vi "Inspect Update Global Variables.vi"(11 "Mode":enum16{"Start", "End"}(ring)) -> ()   [LabVIEW 2019]
uses:
  Common.llb/IVB Variable Data Cluster.ctl
  <vilib>/vision/Image Controls.llb/IMAQ Image.ctl
  Common.llb/IVB Global Variable - Manager Mode.ctl
  Common.llb/IVB Measure ID.ctl
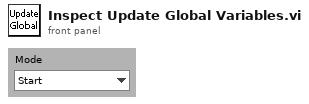
[diagram p1: front panel]
types:
  T1 = typedef "IVB Variable Data Cluster.ctl" = cluster{"String":string, "Numeric":dbl, "Boolean":bool, "Point":cluster{"X":dbl, "Y":dbl}, "Image":T2, "1D String":string[], "1D Numeric":dbl[], "1D Boolean":bool[]}
  T2 = typedef "IMAQ Image.ctl" = refnum<image>
  T3 = typedef "IVB Measure ID.ctl" = cluster{"Step GUID":string, "Result GUID":string, "Index":i32}
  T4 = typedef "IVB Global Variable - Manager Mode.ctl" = enum16{"Init", "Delete User Defined", "Update User Defined", "Get All User Defined", "Get All System", "Set Current Value System", "Set Current Value User Defined", "Add/Update Variable"}
  T5 = enum16{"Reset", "Start Process", "Suspend Process", "Add Elapsed Time", "Get Results"}
  T6 = cluster{"Numeric":dbl, "Boolean":bool, "String":string, "1D Numeric":dbl[], "1D Boolean":bool[], "1D String":string[]}
  T7 = cluster{"Active Time":dbl, "Idle Time":dbl, "Ratio Active/Total":dbl}
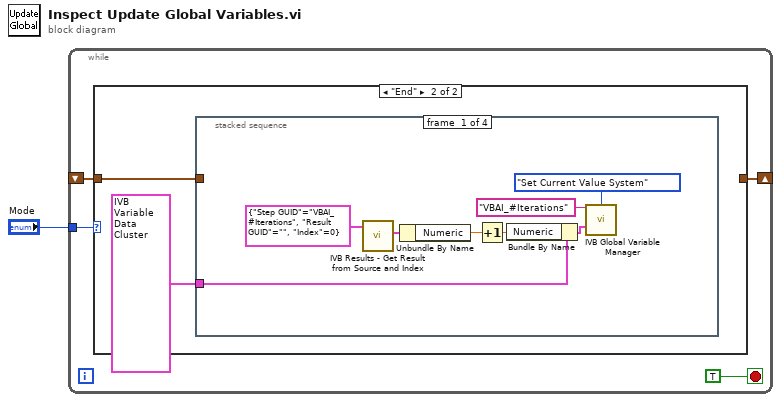
[diagram p0: block diagram]
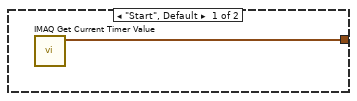
[diagram p2: hidden frame]
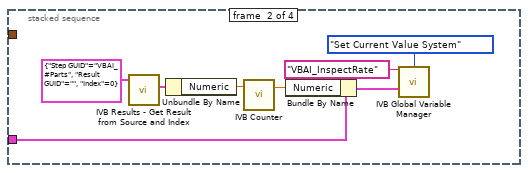
[diagram p3: hidden frame]
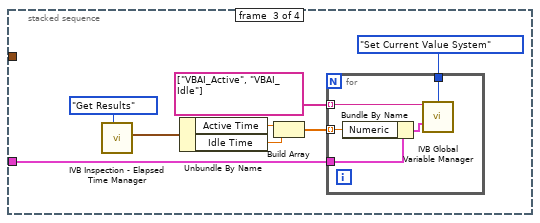
[diagram p4: hidden frame]
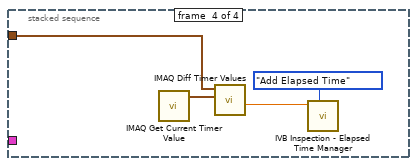
[diagram p5: hidden frame]
diagram:
  n1 = while {
    tunnel: "Mode" -> [w5]
    shift-right: [w4] -> _
    shift-left: _ -> [w3]
    stop <- TRUE stop-if-true
    n2 = case shown="\"End\"" w5 {
      tunnel: [w6 _] -> w4
      tunnel: w3 -> [_ w8]
      frame "Start", Default {
        n3 = call "IMAQ Get Current Timer Value.vi"() -> ("Current Timer Value"=w6:cluster{i32, i32})  [unwired: 10 in, 1 out]
      }
      frame "End" {
        n4 = stacked-sequence {
          tunnel: w8 -> [_ _ _ w38]
          tunnel: T1 {"String"="", "Numeric"=0.0, "Boolean"=FALSE, "Point"={"X"=0.0, "Y"=0.0}, "Image"=refnum, "1D String"=[], "1D Numeric"=[], "1D Boolean"=[]} ("Data In") -> [w13 w22 w25 _]
          frame #0 {
            n5 = call "IVB Results - Get Result from Source and Index.vi"("Measure ID"=T3 {"Step GUID"="VBAI_#Iterations", "Result GUID"="", "Index"=0}) -> ("Result Value"=w9:T6)  [unwired: 6 in, 4 out]
            n6 = Unbundle By Name(w9) -> ("Numeric"=w14:dbl)
            n7 = Increment(x=w14) -> (x+1=w12:dbl)
            n8 = Bundle By Name(cluster=w13, "Numeric"=w12) -> (w11:T1)
            n9 = call "IVB Global Variable Manager.vi"("GUID"="VBAI_#Iterations", "Function"=IVB_Global_Variable_-_Manager_Mode."Set Current Value System", "Data In"=w11) -> ()  [unwired: 11 in, 2 out]
          }
          frame #1 {
            n10 = call "IVB Results - Get Result from Source and Index.vi"("Measure ID"=T3 {"Step GUID"="VBAI_#Parts", "Result GUID"="", "Index"=0}) -> ("Result Value"=w18:T6)  [unwired: 6 in, 4 out]
            n11 = Unbundle By Name(w18) -> ("Numeric"=w17:dbl)
            n12 = call "IVB Counter.vi"("#Parts Inspected"=w17) -> ("Iterations/s"=w21:dbl)  [unwired: 2 in]
            n13 = Bundle By Name(cluster=w22, "Numeric"=w21) -> (w20:T1)
            n14 = call "IVB Global Variable Manager.vi"("GUID"="VBAI_InspectRate", "Function"=IVB_Global_Variable_-_Manager_Mode."Set Current Value System", "Data In"=w20) -> ()  [unwired: 11 in, 2 out]
          }
          frame #2 {
            n15 = call "IVB Inspection - Elapsed Time Manager.vi"("Function"=T5."Get Results") -> ("Total Statistics (s)"=w26:T7)  [unwired: 7 in, 3 out]
            n16 = Unbundle By Name(w26) -> ("Active Time"=w30:dbl, "Idle Time"=w31:dbl)
            n17 = Build Array(w30, w31) -> (w32:dbl[])
            n18 = for {
              tunnel: w32 -> [w34] mode=indexing
              tunnel: string[] ["VBAI_Active", "VBAI_Idle"] -> [w37] mode=indexing
              tunnel: IVB_Global_Variable_-_Manager_Mode."Set Current Value System" ("Function") -> [w36]
              tunnel: w25 -> [w35]
              n19 = Bundle By Name(cluster=w35, "Numeric"=w34) -> (w33:T1)
              n20 = call "IVB Global Variable Manager.vi"("GUID"=w37, "Function"=w36, "Data In"=w33) -> ()  [unwired: 11 in, 2 out]
            }
          }
          frame #3 {
            n21 = call "IMAQ Get Current Timer Value.vi"() -> ("Current Timer Value"=w40:cluster{i32, i32})  [unwired: 10 in, 1 out]
            n22 = call "IMAQ Diff Timer Values.vi"("End Timer Value"=w40, "Start Timer Value"=w38) -> ("Difference (seconds)"=w39:dbl)  [unwired: 6 in, 3 out]
            n23 = call "IVB Inspection - Elapsed Time Manager.vi"("Function"=T5."Add Elapsed Time", "Process Time (s)"=w39) -> ()  [unwired: 6 in, 4 out]
          }
        }
      }
    }
  }
